vi "Setresponse notifier.vi"(8 "error in (no error)":errorcluster, 10 "response notifier":refnum<notifier>, 11 "reference in":refnum<class "UE_slave.lvclass">) -> (0 "error out":errorcluster, 3 "reference out":refnum<class "UE_slave.lvclass">)   [LabVIEW 2019, in "CommandResponse communication.lvlib" / "UE_slave.lvclass"]
uses:
  UE_slave.lvclass
  Status + response + data cluster.ctl
  CommandResponse communication.lvlib
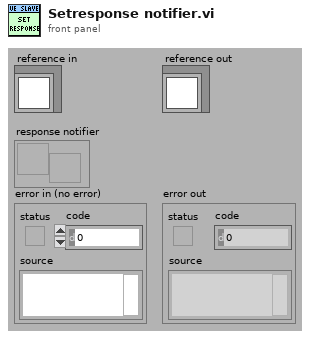
[diagram p1: front panel]
types:
  T1 = typedef "CommandResponse communication.lvlib/UE_slave.lvclass/ObjectAttributesRef.ctl" = refnum<data-value>
  T2 = typedef "CommandResponse communication.lvlib/UE_slave.lvclass/ObjectAttributes.ctl" = cluster{"response notifier":refnum<notifier>}
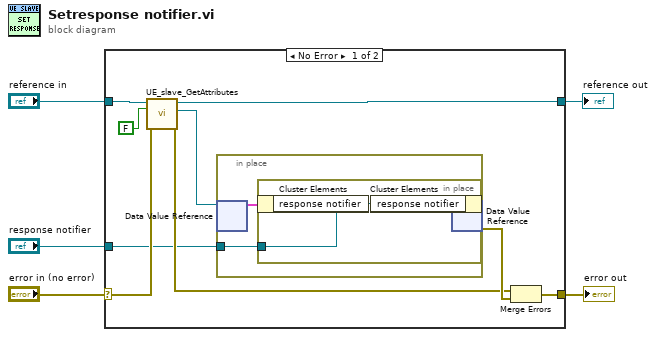
[diagram p0: block diagram]
diagram:
  n1 = case shown="No Error" "error in (no error)" {
    selector: "error in (no error)" -> [w14 w20]
    tunnel: [w8 w20] -> w4
    tunnel: [w13 w19] -> w2
    tunnel: "reference in" -> [w12 w19]
    tunnel: "response notifier" -> [w6 _]
    frame No Error {
      n2 = call "UE_slave_GetAttributes.vi"("error in (no error)"=w14, "return data? (T)"=FALSE, "reference in"=w12) -> ("error out"=w9:errorcluster, "attributes ref"=w7:T1, "reference out"=w13:refnum<class "UE_slave.lvclass">)  [unwired: 5 in, 1 out]
      n3 = in-place {
        in-place-border: w6 -> [w15]
        n4 = in-place-dvr #1(w7) -> (w16:T2)  [unwired: 1 out]
        n5 = in-place {
          in-place-border: w15 -> [w18]
          n6 = in-place-cluster #2(w16) -> ()  [unwired: 1 out]
          n7 = in-place-cluster #2("response notifier"=w18) -> (w17:T2)
        }
        n8 = in-place-dvr #1(w17) -> (w10:errorcluster)  [unwired: 1 out]
      }
      n9 = Merge Errors(w9, w10) -> (w8:errorcluster)
    }
    frame Error {
    }
  }
  "error out" <- w4
  "reference out" <- w2
